vi "main OP500_V2.vi"() -> ()   [LabVIEW 2020]
uses:
  SubVI/OP500ZP_state.ctl
  <userlib>/Alex.vi/FGV.ctl
  <vilib>/QMT/GDataBase for MySQL(tm)/MySQL/public/controls/DateType.ctl
  VG/VG_progressBar.vi
  SubVI/CheminDeBase.vi
  <vilib>/Utility/error.llb/Error Cluster From Error Code.vi
  VG/PN.vi
  VG/PackType.vi
  VG/IS30%.vi
  VG/VG_branche.vi
  VG/Ubatt.vi
  VG/VG_BT3562.vi
  SubVI/OP500ZP_VGConf.vi
  <vilib>/QMT/GDataBase for MySQL(tm)/MySQL/MySQLConnector.lvclass
panel:
  in  "?":bool
  out "N° Révision":u32
  out "IS30% ?":bool
  out "BDD":T1
  out "VISA OUT":T2
  out "progression":u8(slide) scale=0.0..100.0
  out "PN":string
  out "errout 2":errorcluster={"status"=TRUE, "code"=0, "source"="PCAN_CHANNEL ILLEGAL"} caption="errout"
  out "errout":errorcluster caption="sortie d'erreur"
  out "STOP":bool
  out "TOP":string
  out "DRAW":picture
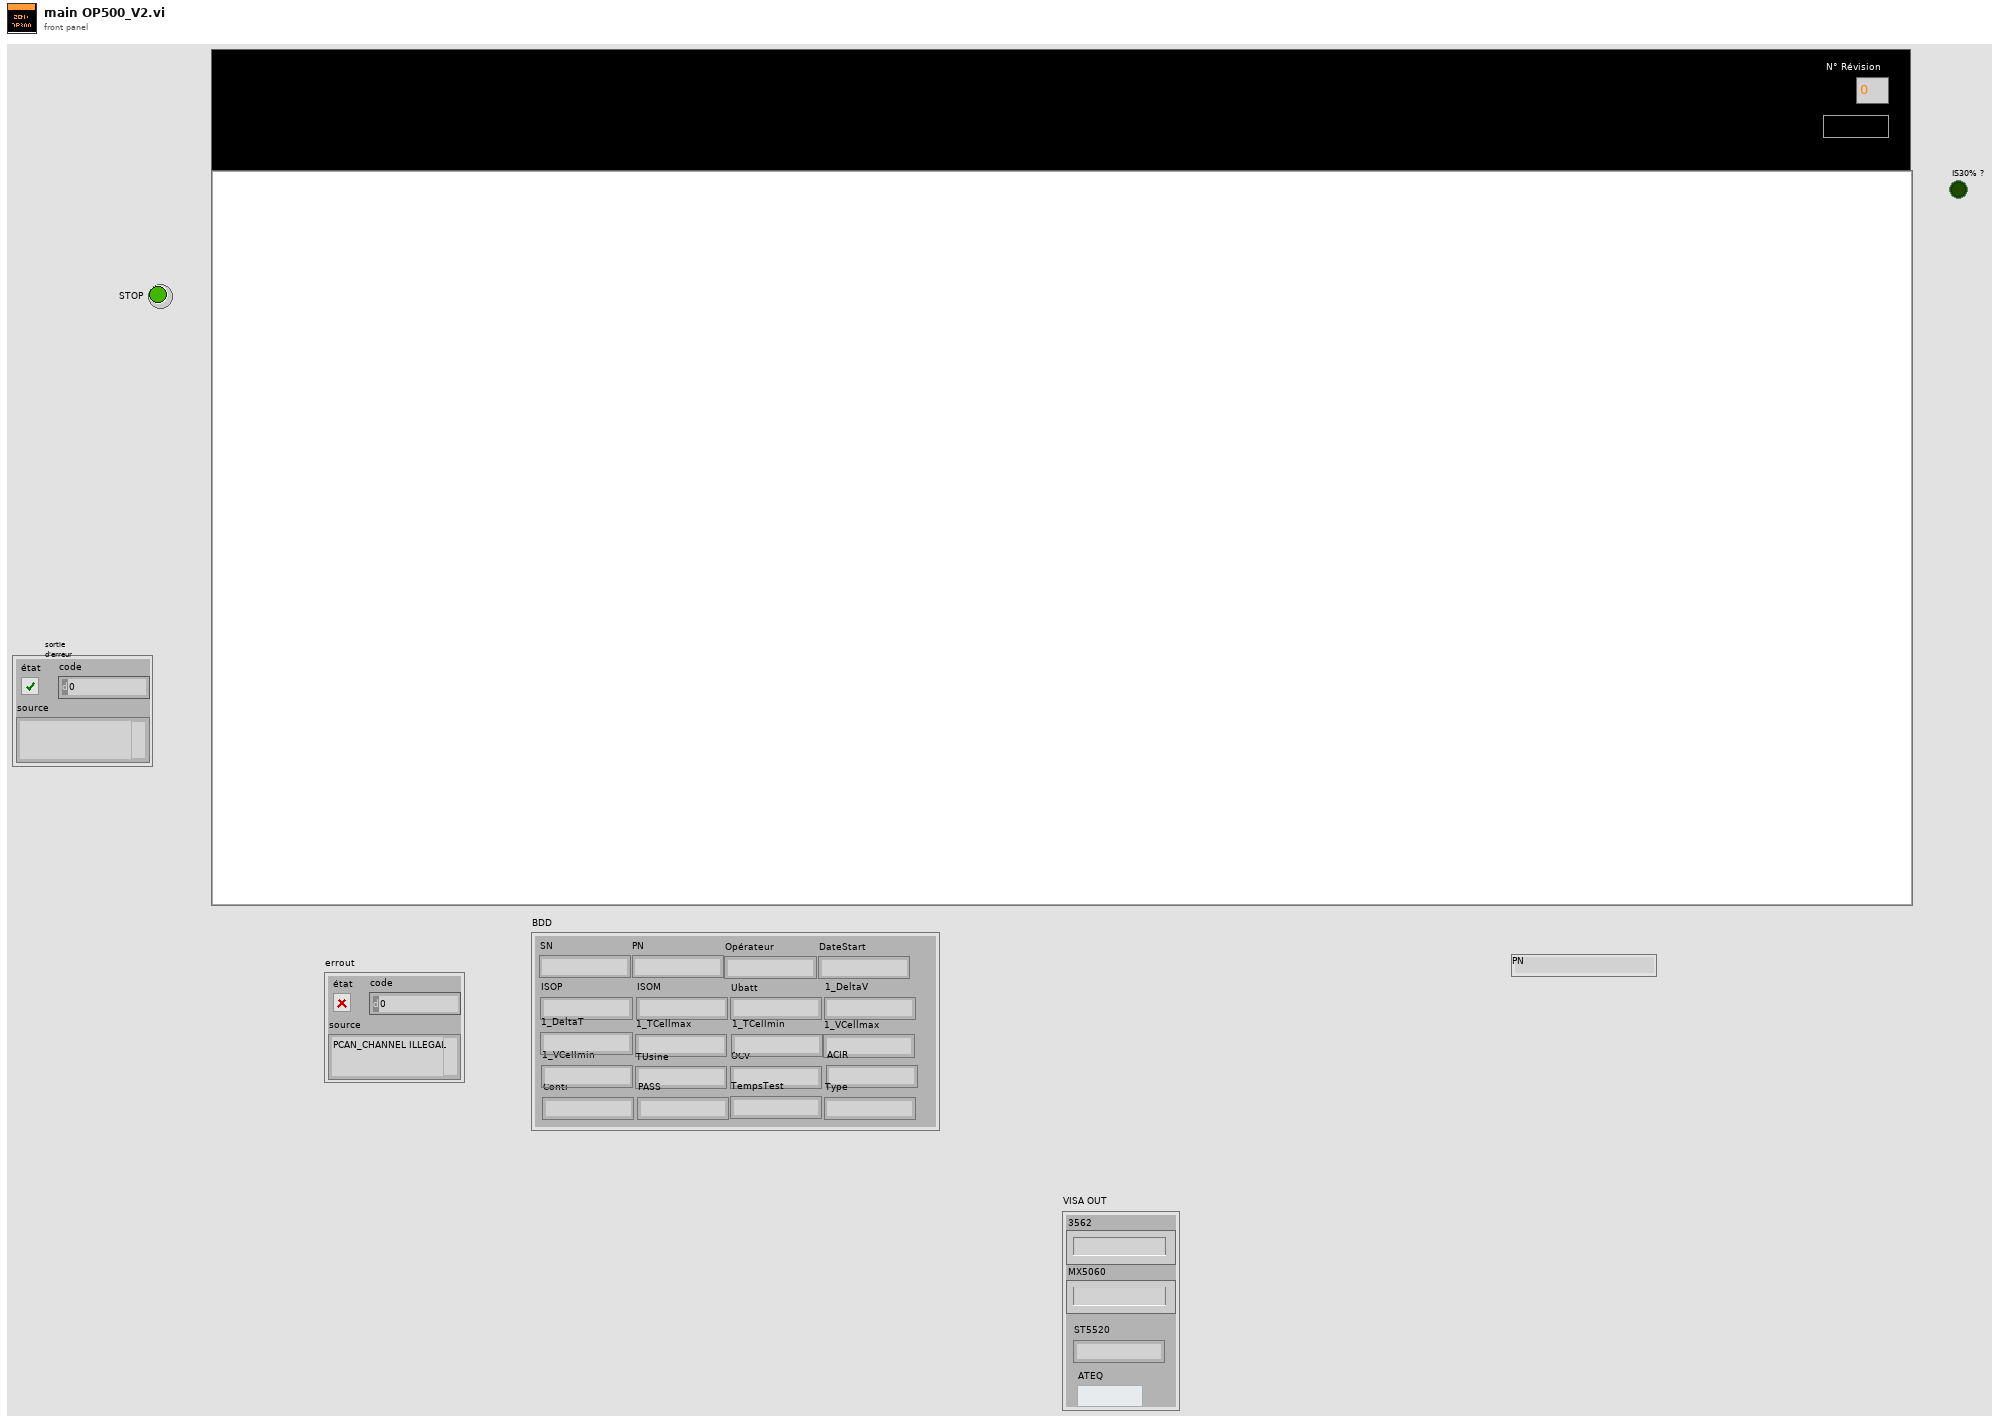
[diagram p1: front panel]
types:
  T1 = cluster{"SN":string, "PN":string, "Opérateur":string, "DateStart":string, "ISOP":string, "ISOM":string, "Ubatt":string, "1_DeltaV":string, "1_DeltaT":string, "1_TCellmax":string, "1_TCellmin":string, "1_VCellmax":string, "1_VCellmin":string, "TUsine":string, "OCV":string, "ACIR":string, "Conti":string, "PASS":string, "TempsTest":string, "Type":string}
  T2 = cluster{"3562":string, "MX5060":string, "ST5520":string, "ATEQ":string}
  T3 = cluster{"PN":string, "Sealing":string, "Opérateur":string, "Conti":string, "OCV":string, "ISOP":string, "ISOM":string, "1_TCellmin":string, "1_TCellmax":string, "1_VCellmin":string, "1_VCellmax":string, "1_Nbmodule":string, "2_TCellmin":string, "2_TCellmax":string, "2_VCellmin":string, "2_VCellmax":string, "2_Nbmodule":string, "Résultat final":string, "Résultat final 2":string, "Résultat final 3":string}
  T4 = cluster{"3562":string, "MX5060":string, "ST5520":string, string}
  T5 = typedef "OP500ZP_state.ctl" = enum16{"Null", "Demarrage", "Init", "Scan", "Iso", "Softs", "MCU", "OCVACIR", "Conti", "DTC", "DataDyn", "DataDyn2", "Crash", "Next", "Comext"}
  T6 = typedef "FGV.ctl" = enum16{"GET", "SET", "RAZ"}
  T7 = typedef "MySQLVIEW.lvlib/MySQLConnector.lvclass/DateType.ctl" = enum16{"DATETIME", "DATE", "TIMESTAMP", "TIME", "YEAR (2 digits)", "YEAR (4 digits)"}
  T8 = cluster{string, string, string, string, string, string, string, string}
  T9 = typedef "OP500ZP_state.ctl" = enum16{"Null", "Demarrage", "Init", "Scan", "Montage", "Conti", "OCV", "Iso", "Softs", "Vpack", "DataDyn", "Dessouter", "DataDyn2", "Demontage", "Crash", "Next", "Sealing", "Comext"}
  T10 = cluster{"Chaîne":string, "Chaîne":string, "Chaîne":string, "Chaîne":string, "Chaîne":string, "Chaîne":string, "Chaîne":string, "Chaîne 2":string}
  T11 = typedef "imagedata.ctl" = cluster{"image type":i32, "image depth":i32, "image":u8[], "mask":u8[], "colors":u32[], "Rectangle":cluster{"left":i16, "top":i16, "right":i16, "bottom":i16}}
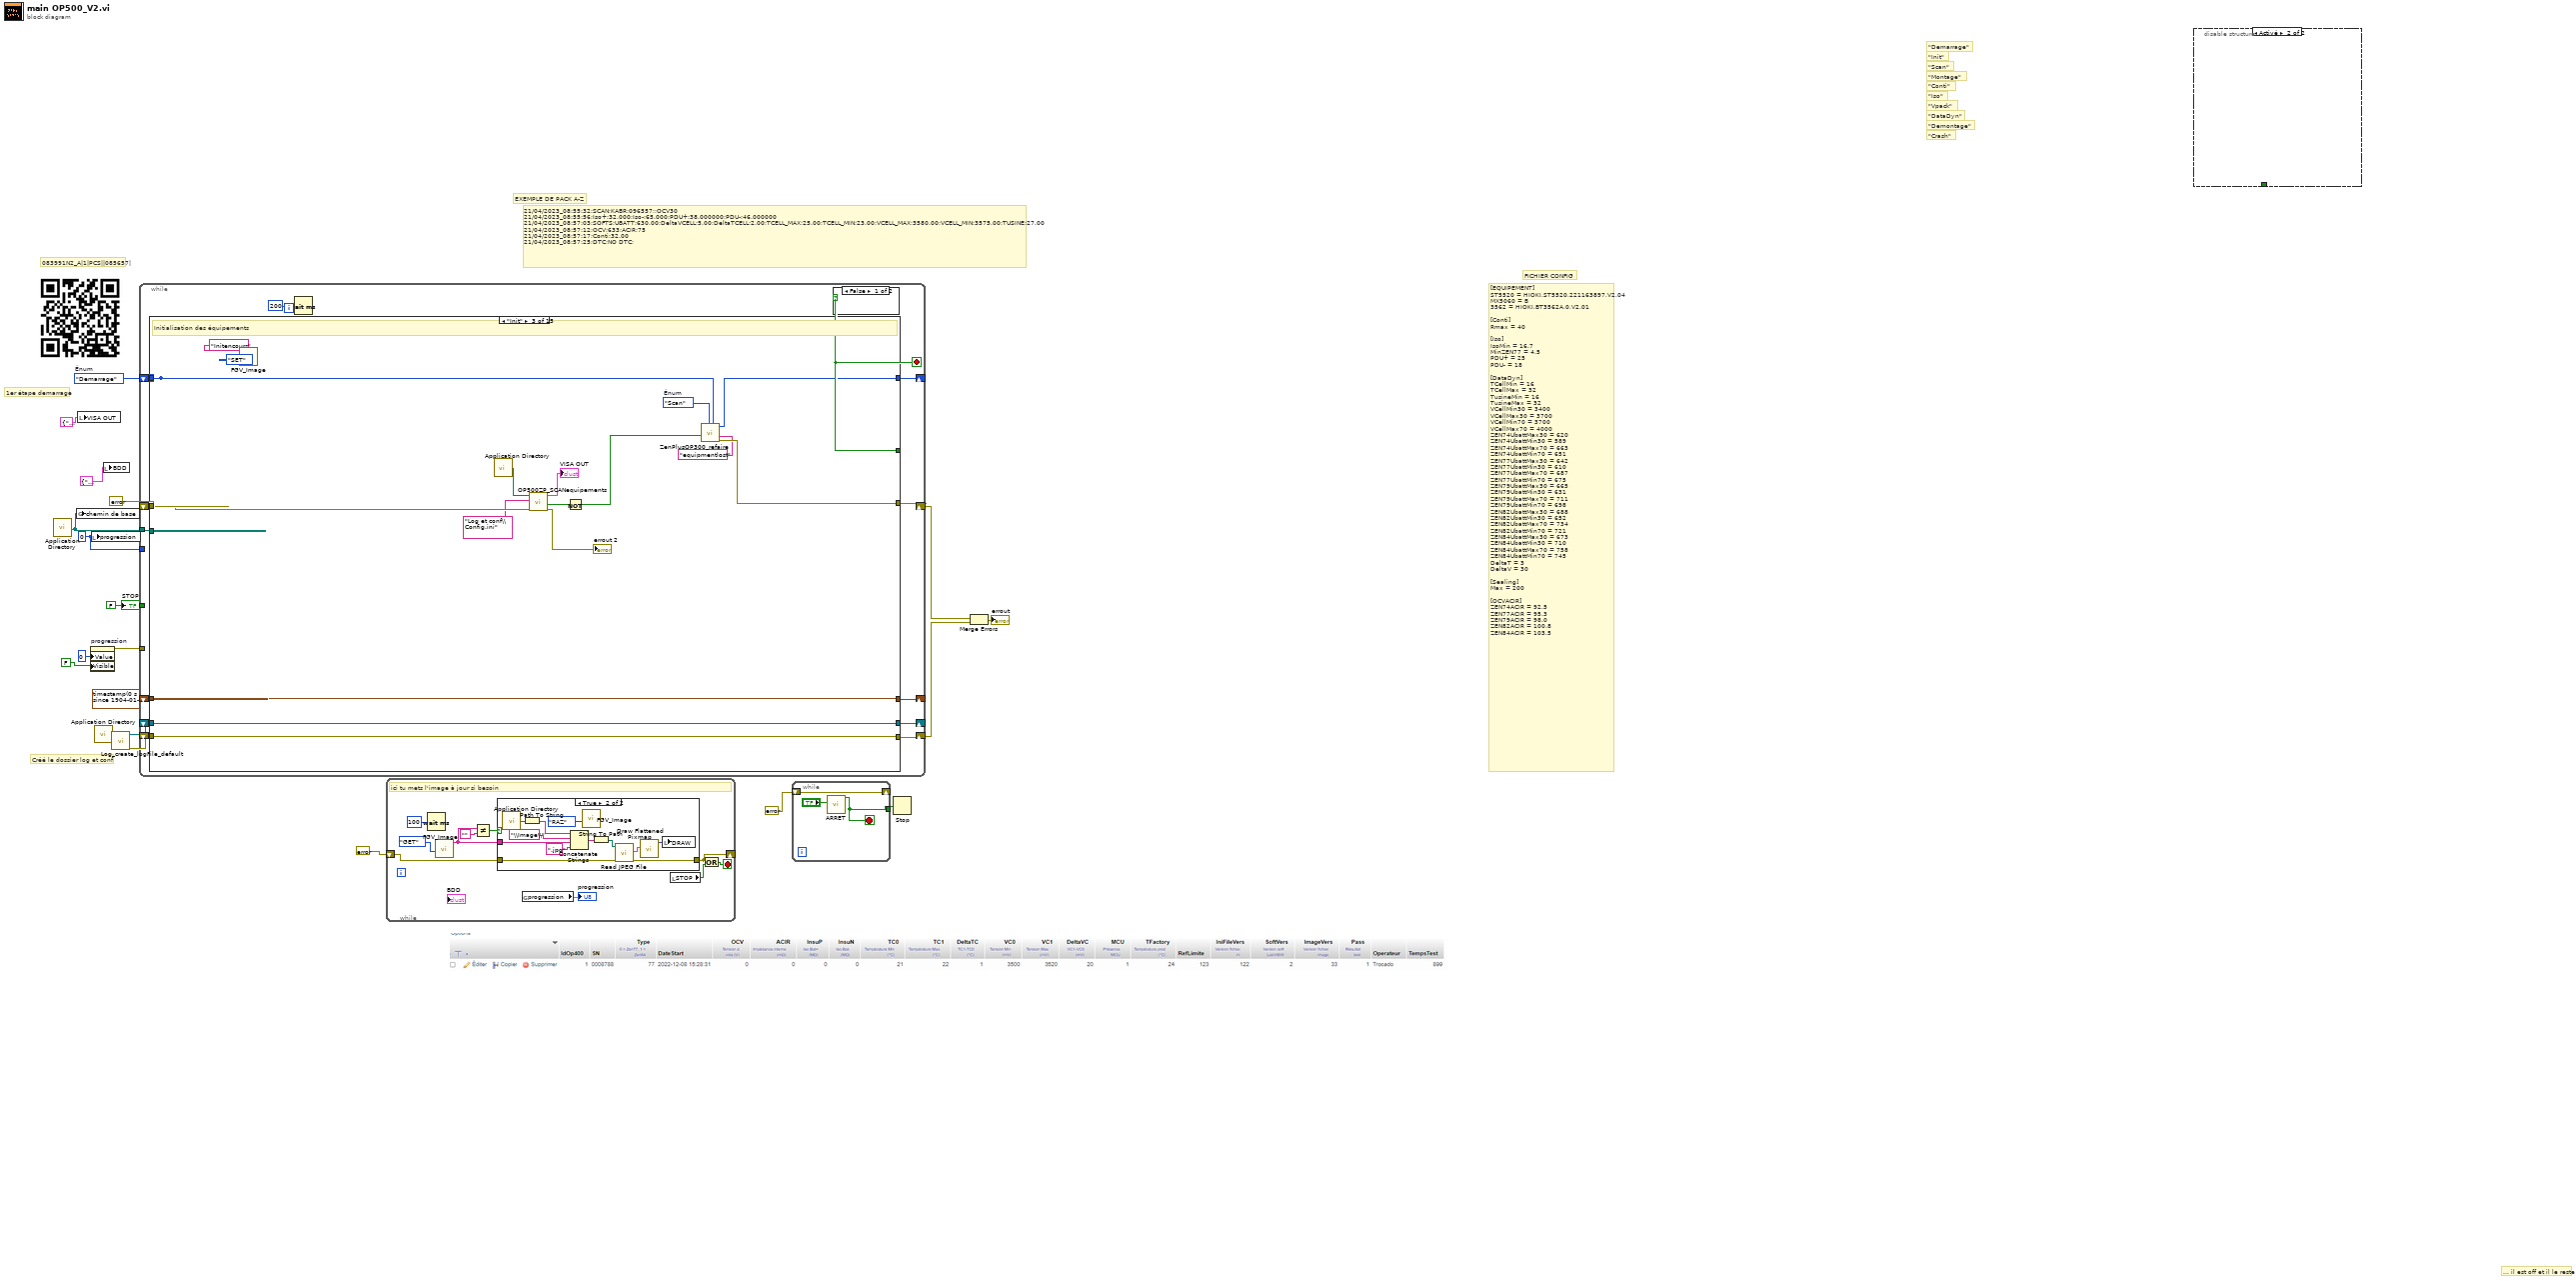
[diagram p0: block diagram]
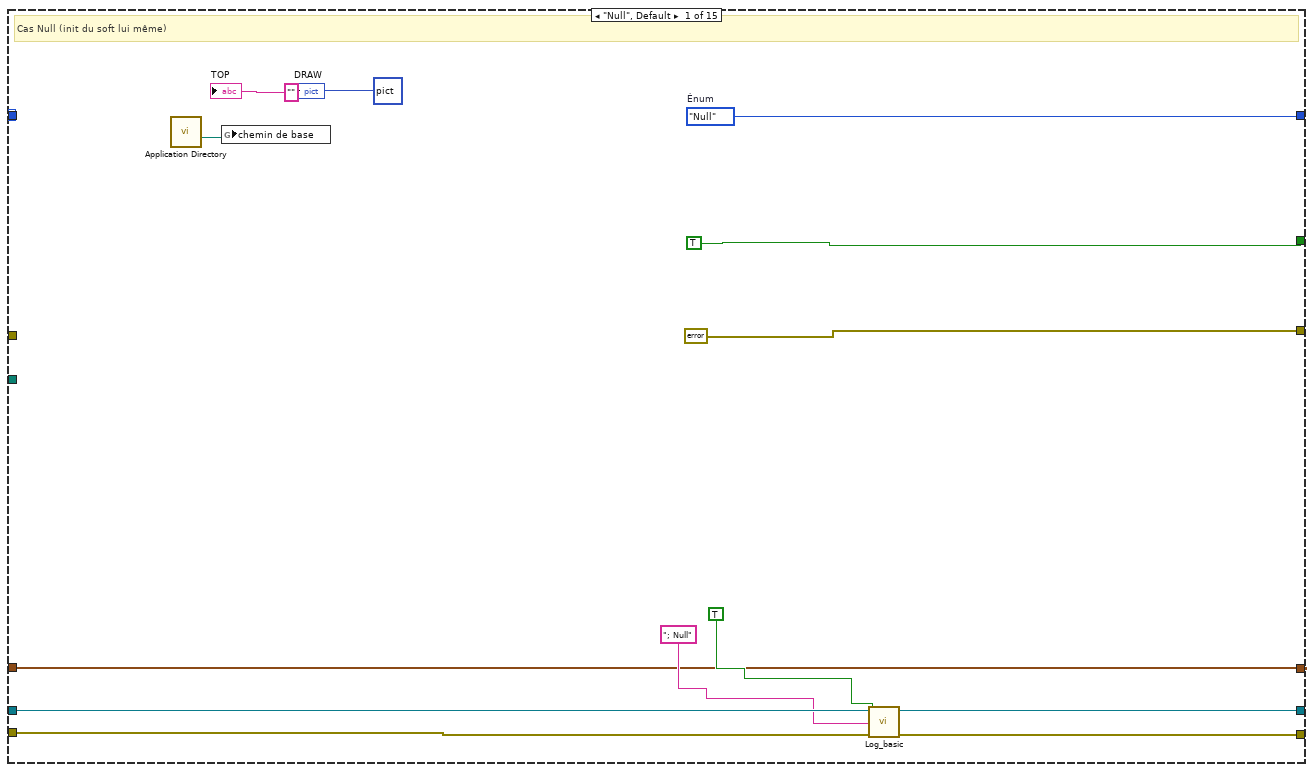
[diagram p2: hidden frame]
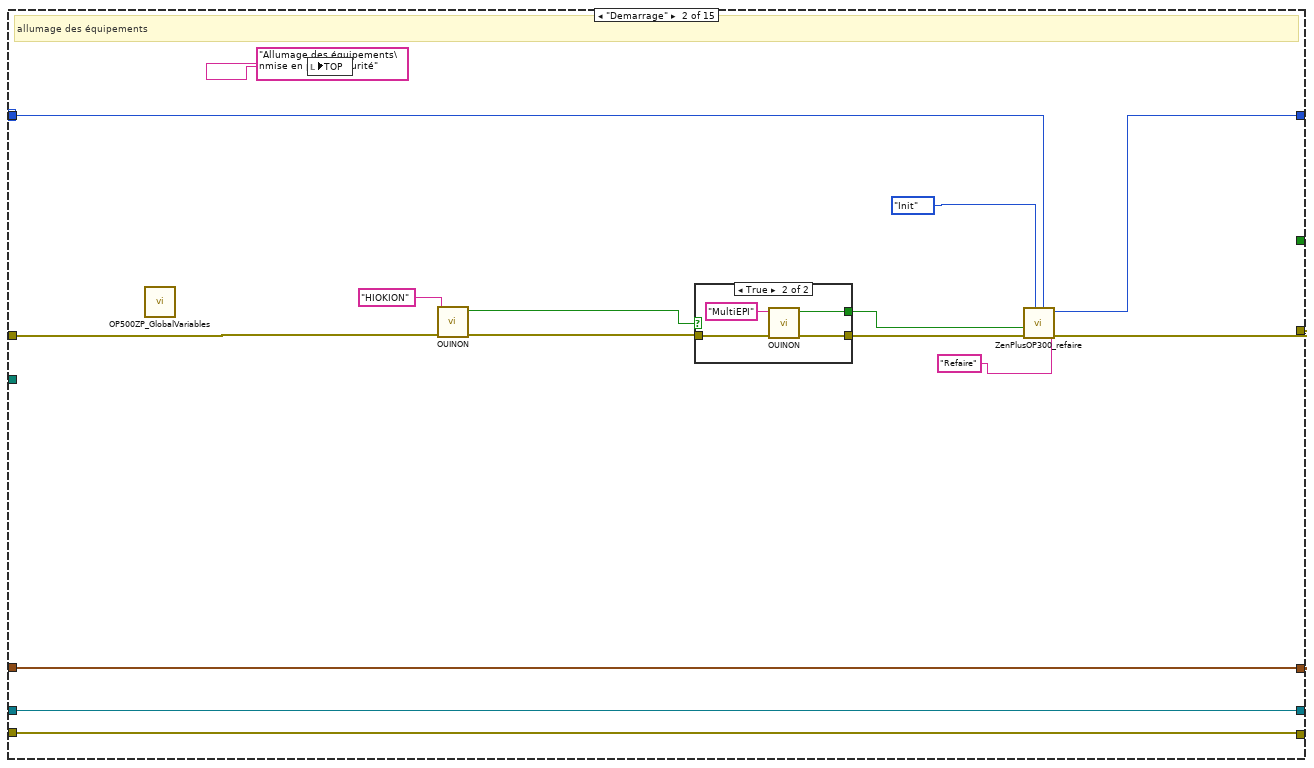
[diagram p3: hidden frame]
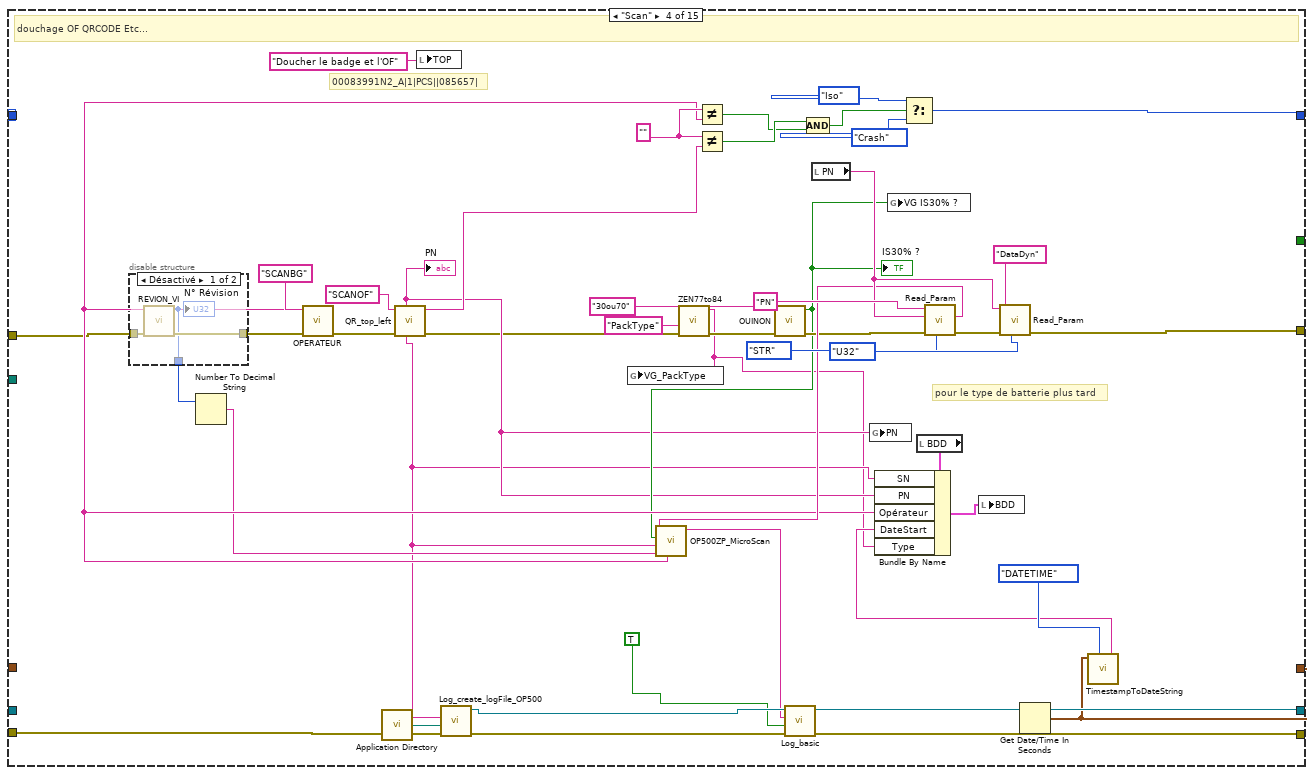
[diagram p5: hidden frame]
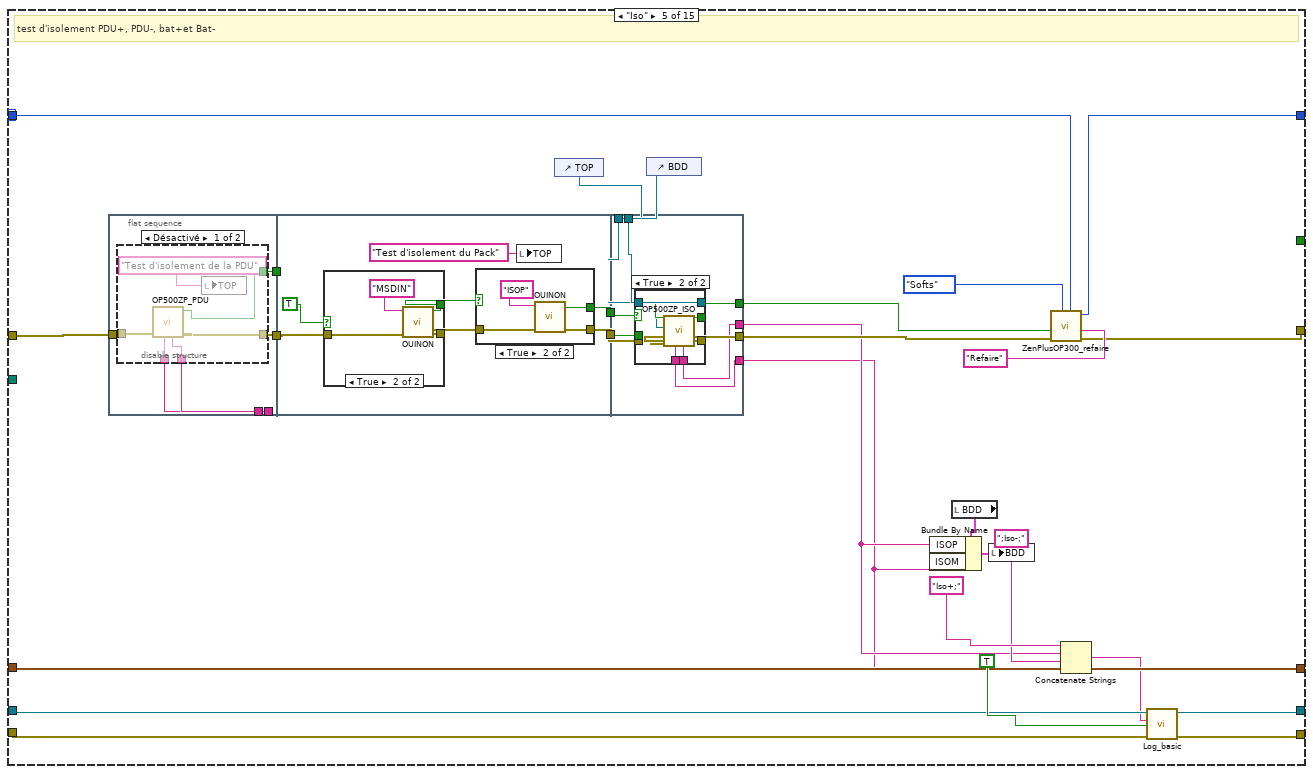
[diagram p7: hidden frame]
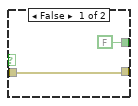
[diagram p9: hidden frame]
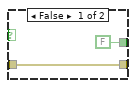
[diagram p10: hidden frame]
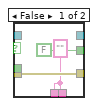
[diagram p11: hidden frame]
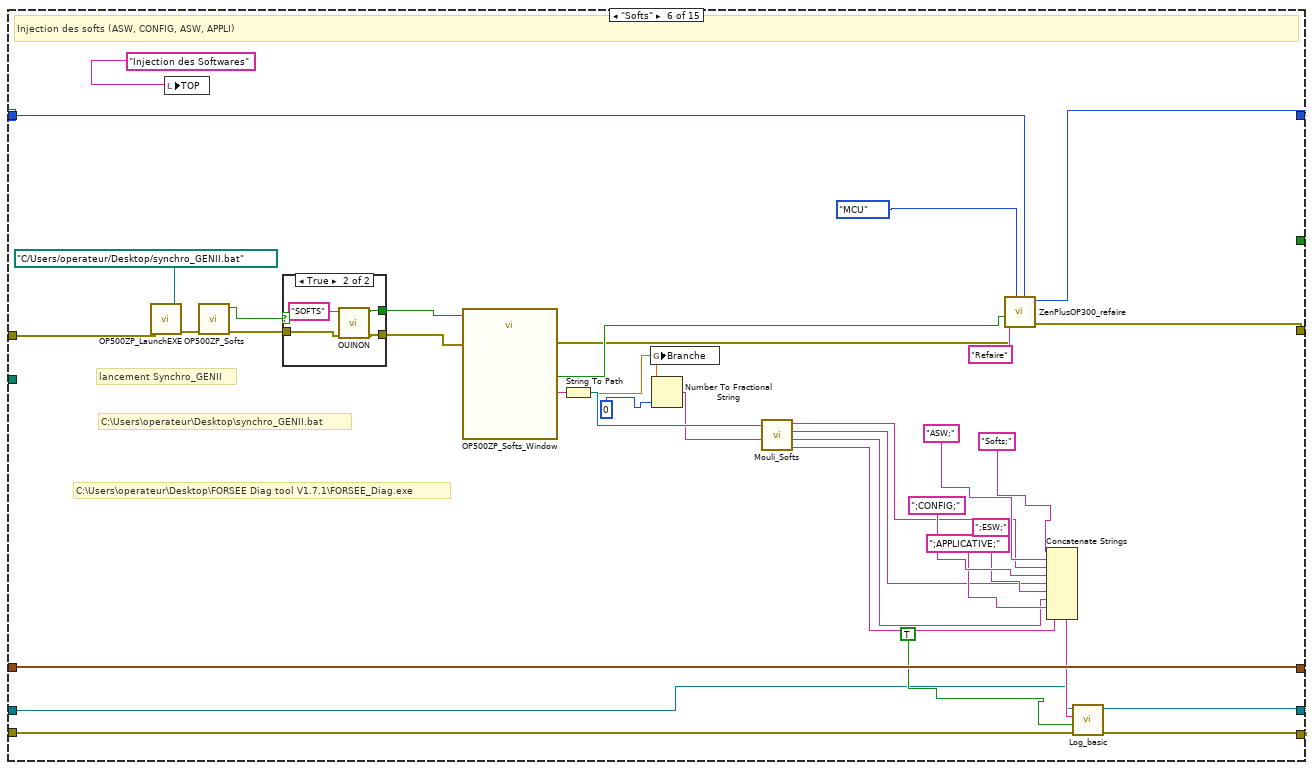
[diagram p12: hidden frame]
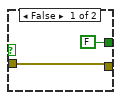
[diagram p13: hidden frame]
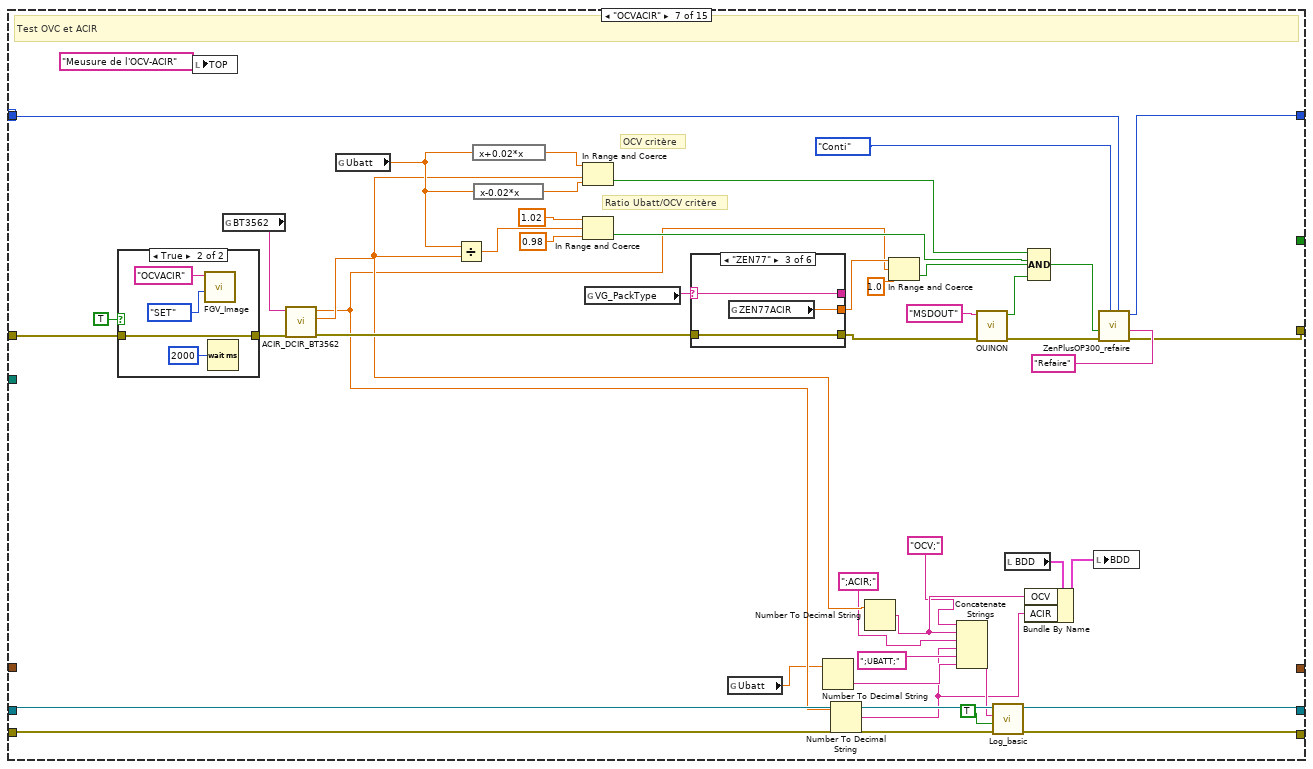
[diagram p14: hidden frame]
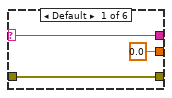
[diagram p16: hidden frame]
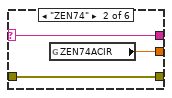
[diagram p17: hidden frame]
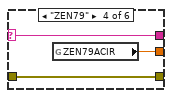
[diagram p18: hidden frame]
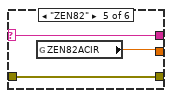
[diagram p19: hidden frame]
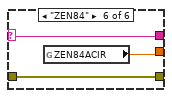
[diagram p20: hidden frame]
diagram:
  w10 = u8 0 ("progression")
  w5 = OP500ZP_state."Demarrage"  # Énum
  w16 = FALSE ("STOP")
  # "083991N2_A|1|PCS||085657|"
  # "EXEMPLE DE PACK A-Z"
  # "21/04/2023_08:55:32;SCAN;KABR;096557;;OCV30\n21/04/2023_08:55:56;Iso+;32.000;Iso-;65.000;PDU+;38.000000;PDU-;46.000000\n21/04/2023_08:57:03;SOFTS;UBATT;630.00;DeltaVCELL;5.00;DeltaTCELL;2.00;TCELL_MAX;25.00;TCELL_MIN;23.00;VCELL_MAX;3580.00;VCELL_MIN;3575.00;TUSINE;27.00\n21/04/2023_08:57:12;OCV;633;ACIR;75\n21/04/2023_08:57:17;Conti;32.00\n21/04/2023_08:57:25;DTC;NO DTC;"
  # "FICHIER CONFIG"
  # "[EQUIPEMENT]\nST5520 = HIOKI,ST5520,221163897,V2.04\t\nMX5060 = B\n3562 = HIOKI,BT3562A,0,V2.01\n\n[Conti]\nRmax = 40\n\n[Iso]\nIsoMin = 16.7\nMinZEN77 = 4.5\nPDU+ = 25\nPDU- = 18\n\n[DataDyn]\nTCellMin = 16\nTCellMax = 32\nTusineMin = 16\nTusineMax = 32\nVCellMin30 = 3400\nVCellMax30 = 3700\nVCellMin70 = 3700\nVCellMax70 = 4000\nZEN74UbattMax30 = 620\nZEN74UbattMin30 = 589\nZEN74UbattMax70 = 663\nZEN74UbattMin70 = 651\nZEN77UbattMax30 = 642\nZEN77UbattMin30 = 610\nZEN77UbattMax70 = 687\nZEN77UbattMin70 = 675\nZEN79UbattMax30 = 665\nZEN79UbattMin30 = 631\nZEN79UbattMax70 = 711\nZEN79UbattMin70 = 698\nZEN82UbattMax30 = 688\nZEN82UbattMin30 = 652\nZEN82UbattMax70 = 734\nZEN82UbattMin70 = 721\nZEN84UbattMax30 = 673\nZEN84UbattMin30 = 710\nZEN84UbattMax70 = 758\nZEN84UbattMin70 = 745\nDeltaT = 3\nDeltaV = 30\n\n[Sealing]\nMax = 200\n\n[OCVACIR]\nZEN74ACIR = 92.5\nZEN77ACIR = 95.3\nZEN79ACIR = 98.0\nZEN82ACIR = 100.8\nZEN84ACIR = 103.5"
  # "Créé le dossier log et conf"
  # "1er étape demarrage"
  # "\"Crash\""
  # "\"Demontage\""
  # "\"DataDyn\""
  # "\"Iso\""
  # "\"Montage\""
  # "\"Scan\""
  # "\"Init\""
  # "\"Demarrage\""
  # "\"Conti\""
  # "\"Vpack\""
  # "... il est off et il le reste"
  n1 = call <vilib>:"Application Directory.vi"() -> ("Application Directory"=w15:path)
  n2 = global write "CheminDeBase.vi" "chemin de base"(w15) -> ()
  n3 = local write "VISA OUT"(T4 {"3562"="", "MX5060"="", "ST5520"="", ""} ("VISA OUT")) -> ()
  n4 = property on="progression" class="Slide (strict)"("Value"=u8 0 ("progression"), "Visible"=FALSE) -> (error out=w8:errorcluster)  [unwired: 2 in, 1 out]
  n5 = local write "progression"(w10) -> ()
  n6 = call <vilib>:"Application Directory.vi"() -> ("Application Directory"=w13:path)
  n7 = local write "BDD"(T3 {"PN"="0", "Sealing"="0", "Opérateur"="0", "Conti"="0", "OCV"="0", "ISOP"="0", "ISOM"="0", "1_TCellmin"="0", "1_TCellmax"="0", "1_VCellmin"="0", "1_VCellmax"="0", "1_Nbmodule"="0", "2_TCellmin"="0", "2_TCellmax"="0", "2_VCellmin"="0", "2_VCellmax"="0", "2_Nbmodule"="0", "Résultat final"="0", "Résultat final 2"="0", "Résultat final 3"="0"} ("Cluster")) -> ()
  n8 = call <userlib>:"Log_create_logFile_default.vi"("appdir"=w13) -> ("errout"=w14:errorcluster, "Fichier à flux d'octets en sortie"=w17:refnum<file>)  [unwired: 9 in]
  n9 = while {
    shift-right: [w32] -> w19
    shift-left: errorcluster {"status"=FALSE, "code"=0, "source"=""} ("error out") -> [w24]
    shift-right: [w28] -> w18
    shift-left: w14 -> [w31]
    shift-right: [w29] -> _
    shift-left: w17 -> [w30]
    tunnel: w15 -> [w27]
    tunnel: w16 -> [_]
    shift-right: [w25] -> _
    shift-left: timestamp(0 s since 1904-01-01) ("seconds since 1Jan1904") -> [w26]
    tunnel: w10 -> [_]
    tunnel: w8 -> [_]
    shift-right: [w23] -> _
    shift-left: w5 -> [w22]
    stop <- w21 stop-if-true
    n10 = case shown="\"Init\"" w22 {
      selector: w22 -> [_ w50 w80 _ _ w239 w291 w342 w395 _ w469 _ _ w594 w694]
      tunnel: w24 -> [_ w60 w74 w93 w146 w237 w255 w323 w376 w439 w461 w523 w555 w591 w691]
      tunnel: [errorcluster {"status"=FALSE, "code"=0, "source"=""} ("errin") w51 w81 w115 w144 w241 w290 w343 w396 w443 w462 w522 w558 w593 w696] -> w32
      tunnel: w31 -> [w42 w54 w84 w128 w159 w230 w287 w349 w389 w448 w465 w545 w578 w597 w703]
      tunnel: w30 -> [w43 w61 w83 _ w158 w228 w289 w348 w387 w447 w467 w546 w579 w596 w702]
      tunnel: [w40 w61 w83 w130 w157 w227 w288 w347 w386 w446 w463 _ _ w588 w700] -> w29
      tunnel: [w41 w54 w84 w131 w160 w229 w286 w346 w388 w445 w464 w524 w556 w595 w701] -> w28
      tunnel: [TRUE _ _ _ _ _ _ _ _ _ _ w547 _ _ _] -> w21
      tunnel: w27 -> [_ _ _ _ _ _ _ _ _ _ w468 _ _ w592 _]
      tunnel: w26 -> [w37 w59 w82 _ w156 w245 _ w345 w384 w427 w466 _ _ w589 w699]
      tunnel: [w37 w59 w82 w88 w156 w245 _ w345 w384 w427 w466 _ _ w590 w699] -> w25
      tunnel: [w34 w48 w78 w94 w141 w240 w275 w336 w393 w425 w460 OP500ZP_state."Crash" w557 w587 w693] -> w23
      tunnel: w22 -> [_ _ _ _ w142 _ _ _ _ _ _ _ _ _ _]
      frame "Null", Default {
        w34 = OP500ZP_state."Null"  # Énum
        # "Cas Null (init du soft lui même)"
        n11 = call <vilib>:"Application Directory.vi"() -> ("Application Directory"=w46:path)
        n12 = global write "CheminDeBase.vi" "chemin de base"(w46) -> ()
        n13 = call <userlib>:"Log_basic.vi"("errin"=w42, "date?"=TRUE, "chaîne"="; Null", "in"=w43) -> ("sortie d'erreur"=w41:errorcluster, "refnum en sortie"=w40:refnum<file>)  [unwired: 6 in]
        "DRAW" <- picture data[5B] ("DRAW")
        "TOP" <- "" ("TOP")
      }
      frame "Demarrage" {
        # "allumage des équipements"
        n14 = call "OP500ZP_GlobalVariables.vi"() -> ()  [unwired: 12 in]
        n15 = local write "TOP"("Allumage des équipements\nmise en place sécurité" ("TOP")) -> ()
        n16 = call "OUINON.vi"("errin"=w60, "image"="HIOKION") -> ("error out"=w55:errorcluster, "OUI/NON"=w56:bool)  [unwired: 8 in]
        n17 = case shown="True" w56 {
          selector: w56 -> [w63 _]
          tunnel: [w63 w67] -> w47
          tunnel: [w62 w66] -> w52
          tunnel: w55 -> [w62 w64]
          frame False {
          }
          frame True {
            n18 = call "OUINON.vi"("errin"=w64, "image"="MultiEPI" ("IN")) -> ("error out"=w66:errorcluster, "OUI/NON"=w67:bool)  [unwired: 8 in]
          }
        }
        n19 = call "ZenPlusOP300_refaire.vi"("image"="Refaire", "refaire"=w50, "casOK"=OP500ZP_state."Init", "errin"=w52, "test ok ?"=w47) -> ("errout"=w51:errorcluster, "Next"=w48:T5)  [unwired: 5 in]
      }
      frame "Init" {
        w77 = OP500ZP_state."Scan"  # Énum
        # "Initialisation des équipements"
        n20 = call <userlib>:"FGV_Image.vi"("Énum"=FGV."SET", "IN"="Initencours") -> ()  [unwired: 9 in, 1 out]
        n21 = call <vilib>:"Application Directory.vi"() -> ("Application Directory"=w72:path)
        n22 = call "OP500ZP_SCANequipements.vi"("Errin"=w74, "Chaîne"="Log et conf\\Config.ini", "pathin"=w72) -> ("ERROUT"=→"errout 2":errorcluster, "KO?"=w69:bool, "VISA OUT"=→"VISA OUT":T2)  [unwired: 6 in]
        n23 = Not(x=w69) -> (.not. x?=w68:bool)
        n24 = call "ZenPlusOP300_refaire.vi"("image"="equipmentlost", "refaire"=w80, "casOK"=w77, "test ok ?"=w68) -> ("errout"=w81:errorcluster, "Next"=w78:T5)  [unwired: 6 in]
      }
      frame "Scan" {
        w123 = "" ("x")
        # "pour le type de batterie plus tard"
        # "00083991N2_A|1|PCS||085657|"
        # "douchage OF QRCODE Etc..."
        n25 = disable-structure shown="Désactivé" {
          disable-tunnel: w93 -> [w134 _]
          disable-tunnel: [w133 _] -> w92
          disable-tunnel: [w132 _] -> w91
          frame Disabled {
            n26 = call "REVION_VI.vi"("ERRIN"=w134) -> ("ERROUT"=w133:errorcluster, "N° Révision"=w132:u32)  [unwired: 9 in]
            "N° Révision" <- w132
          }
          frame Enabled {
          }
        }
        n27 = Number To Decimal String(number=w91) -> (decimal integer string=w90:string)  [unwired: 1 in]
        n28 = call <userlib>:"OPERATEUR.vi"("errin"=w92, "IN"="SCANBG") -> ("error out"=w120:errorcluster, "Dataout"=w102:string)  [unwired: 8 in]
        n29 = call <vilib>:"Application Directory.vi"() -> ("Application Directory"=w129:path)
        n30 = call "QR_top_left.vi"("errin"=w120, "image"="SCANOF") -> ("error out"=w97:errorcluster, "Réponse"=w118:string, "SN"=w89:string, "PN"=w98:string)  [unwired: 5 in, 1 out]
        "PN" <- w98
        n31 = local write "TOP"("Doucher le badge et l'OF" ("TOP")) -> ()
        n32 = call "Log_create_logFile_OP500.vi"("errin"=w128, "toute l'expression"=w89, "Application Directory"=w129) -> ("sortie d'erreur"=w126:errorcluster, "Fichier à flux d'octets en sortie"=w127:refnum<file>)  [unwired: 7 in]
        n33 = call <userlib>:"ZEN77to84.vi"("errin"=w97, "image"="PackType") -> ("error out"=w96:errorcluster, "Réponse"=w85:string)  [unwired: 8 in]
        n34 = global write "PackType.vi" "VG_PackType"(w85) -> ()
        n35 = Not Equal?(x=w123, y=w102) -> (x != y?=w121:bool)
        n36 = Not Equal?(x=w123, y=w118) -> (x != y?=w122:bool)
        n37 = call "OUINON.vi"("errin"=w96, "image"="30ou70") -> ("error out"=w100:errorcluster, "OUI/NON"=w99:bool)  [unwired: 8 in]
        "IS30% ?" <- w99
        n38 = Compound Arithmetic op=AND ("Opérateur arithmétique")(w122, w121) -> (w108:bool)
        n39 = local read "PN"() -> (w111:string)
        n40 = global write "PN.vi" "PN"(w98) -> ()
        n41 = global write "IS30%.vi" "VG IS30% ?"(w99) -> ()
        n42 = Select ("Sélectionner")(t=OP500ZP_state."Iso" ("Énum"), s=w108, f=OP500ZP_state."Crash" ("cas faux")) -> (s? t:f=w94:T5)
        n43 = local read "BDD"() -> (w104:T1)
        n44 = call <userlib>:"Read_Param.vi"("Énum"=enum16{"STR", "DBL", "U32"}."STR", "errin"=w100, "section"=w111, "key"="PN") -> ("error out"=w114:errorcluster, "str"=w110:string)  [unwired: 3 in, 3 out]
        n45 = call "OP500ZP_MicroScan.vi"("Dataout"=w102, "Rev"=w90, "SN"=w89, "Oui"=w99, "str"=w110) -> ("Chaîne"=w125:string)  [unwired: 6 in]
        n46 = call <userlib>:"Log_basic.vi"("errin"=w126, "date?"=TRUE, "chaîne"=w125, "in"=w127) -> ("sortie d'erreur"=w131:errorcluster, "refnum en sortie"=w130:refnum<file>)  [unwired: 6 in]
        n47 = call <userlib>:"Read_Param.vi"("Énum"=enum16{"STR", "DBL", "U32"}."U32", "errin"=w114, "section"="DataDyn", "key"=w111) -> ("error out"=w115:errorcluster)  [unwired: 3 in, 4 out]
        n48 = Get Date/Time In Seconds() -> (seconds since 1Jan1904=w88:timestamp)
        n49 = call <vilib>:"TimestampToDateString.vi"("dateType"=DateType."DATETIME", "timestamp in"=w88) -> ("dateString"=w86:string)  [unwired: 8 in, 1 out]
        n50 = Bundle By Name(cluster=w104, "SN"=w89, "PN"=w98, "Opérateur"=w102, "DateStart"=w86, "Type"=w85) -> (w103:T1)
        n51 = local write "BDD"(w103) -> ()
      }
      frame "Iso" {
        # "test d'isolement PDU+, PDU-, bat+et Bat-"
        n52 = flat-sequence {
          tunnel: [w164] -> w148
          tunnel: [w165] -> w147
          tunnel: w146 -> [w166]
          tunnel: [w163] -> _
          tunnel: [w162] -> _
          tunnel: [w179] -> w150
          tunnel: [w178] -> w149
          tunnel: w148 -> [_]
          tunnel: w147 -> [w173]
          tunnel: [w199] -> w140
          tunnel: [w192] -> w135
          tunnel: [w193] -> w136
          tunnel: w152 -> [w197]
          tunnel: w151 -> [w196]
          tunnel: w150 -> [w198]
          tunnel: w149 -> [w195]
          tunnel: [w194] -> w139
          frame #0 {
            n53 = disable-structure shown="Désactivé" {
              disable-tunnel: w166 -> [w172 _]
              disable-tunnel: [w171 _] -> w165
              disable-tunnel: [w170 _] -> w164
              disable-tunnel: [w169 _] -> w163
              disable-tunnel: [w168 _] -> w162
              frame Disabled {
                n54 = call "OP500ZP_PDU.vi"("errin"=w172) -> ("errout"=w171:errorcluster, "PASS?"=w170:bool, "ISO_PDU-"=w169:string, "ISO_PDU+"=w168:string)  [unwired: 7 in]
                n55 = local write "TOP"("Test d'isolement de la PDU" ("TOP")) -> ()
              }
              frame Enabled {
              }
            }
          }
          frame #1 {
            n56 = case shown="True" TRUE {
              tunnel: w173 -> [w181 w185]
              tunnel: [w181 w184] -> w177
              tunnel: [FALSE ("OUI/NON") w182] -> w175
              frame False {
              }
              frame True {
                n57 = call "OUINON.vi"("errin"=w185, "image"="MSDIN") -> ("error out"=w184:errorcluster, "OUI/NON"=w182:bool)  [unwired: 8 in]
              }
            }
            n58 = case shown="True" w175 {
              tunnel: [w186 w191] -> w179
              tunnel: [FALSE ("OUI/NON") w190] -> w178
              tunnel: w177 -> [w186 w188]
              frame False {
              }
              frame True {
                n59 = call "OUINON.vi"("errin"=w188, "image"="ISOP" ("IN")) -> ("error out"=w191:errorcluster, "OUI/NON"=w190:bool)  [unwired: 8 in]
              }
            }
            n60 = local write "TOP"("Test d'isolement du Pack" ("TOP")) -> ()
          }
          frame #2 {
            n61 = case shown="True" w195 {
              tunnel: [w202 w209] -> w199
              tunnel: w198 -> [w202 w208]
              tunnel: w195 -> [_ w207]
              tunnel: w197 -> [_ _]
              tunnel: w196 -> [_ w206]
              tunnel: [FALSE ("Booléen") w205] -> w194
              tunnel: [w200 w204] -> w193
              tunnel: [w200 w203] -> w192
              frame False {
                w200 = "" ("Chaîne")
              }
              frame True {
                n62 = call "OP500ZP_ISO.vi"("entrée d'erreur (pas d'erreur)"=w208, "Oui"=w207, "reference en entrée"=w206) -> ("sortie d'erreur"=w209:errorcluster, "Booléen"=w205:bool, "ISOP"=w204:string, "ISOM"=w203:string)  [unwired: 5 in]
              }
            }
          }
        }
        n63 = control-ref of="TOP"() -> (w151:refnum<vi>)
        n64 = control-ref of="BDD"() -> (w152:refnum<vi>)
        n65 = local read "BDD"() -> (w138:T1)
        n66 = Bundle By Name(cluster=w138, "ISOP"=w136, "ISOM"=w135) -> (w137:T1)
        n67 = local write "BDD"(w137) -> ()
        n68 = call "ZenPlusOP300_refaire.vi"("image"="Refaire", "refaire"=w142, "casOK"=OP500ZP_state."Softs", "errin"=w140, "test ok ?"=w139) -> ("errout"=w144:errorcluster, "Next"=w141:T5)  [unwired: 5 in]
        n69 = Concatenate Strings("Iso+;" ("chaîne"), w136, ";Iso-;" ("chaîne"), w135) -> (w153:string)
        n70 = call <userlib>:"Log_basic.vi"("errin"=w159, "date?"=TRUE, "chaîne"=w153, "in"=w158) -> ("sortie d'erreur"=w160:errorcluster, "refnum en sortie"=w157:refnum<file>)  [unwired: 6 in]
      }
      frame "Softs" {
        # "C:\\Users\\operateur\\Desktop\\FORSEE Diag tool V1.7.1\\FORSEE_Diag.exe"
        # "C:\\Users\\operateur\\Desktop\\synchro_GENII.bat"
        # "lancement Synchro_GENII"
        # "Injection des softs (ASW, CONFIG, ASW, APPLI)"
        n71 = call "OP500ZP_LaunchEXE.vi"("errin"=w237, "Application à lancer"=path "C:/Users/operateur/Desktop/synchro_GENII.bat") -> ("error out"=w244:errorcluster)  [unwired: 7 in]
        n72 = local write "TOP"("Injection des Softwares" ("TOP")) -> ()
        n73 = call "OP500ZP_Softs.vi"("errin"=w244) -> ("errout"=w217:errorcluster, "OUI/NON"=w214:bool)  [unwired: 9 in]
        n74 = case shown="True" w214 {
          tunnel: w217 -> [w246 w251]
          tunnel: [w246 w250] -> w216
          tunnel: [FALSE ("OUI/NON") w249] -> w215
          frame False {
          }
          frame True {
            n75 = call "OUINON.vi"("errin"=w251, "image"="SOFTS") -> ("error out"=w250:errorcluster, "OUI/NON"=w249:bool)  [unwired: 8 in]
          }
        }
        n76 = call "OP500ZP_Softs_Window.vi"("Enable"=w215, "error in (no error)"=w216) -> ("Répertoire softs :"=w236:string, "n° Branche"=w212:dbl, "OK"=w213:bool, "error out"=w211:errorcluster)  [unwired: 14 in]
        n77 = String To Path(string=w236) -> (path=w235:path)
        n78 = global write "VG_branche.vi" "Branche"(w212) -> ()
        n79 = Number To Fractional String(number=w212, precision (6)=i16 0 ("précision (6)")) -> (F-format string=w234:string)  [unwired: 2 in]
        n80 = call "Mouli_Softs.vi"("Branche"=w234, "chemin"=w235) -> ("APPL"=w219:string, "ESW"=w220:string, "CONFIG"=w221:string, "ASW"=w222:string)  [unwired: 6 in]
        n81 = call "ZenPlusOP300_refaire.vi"("image"="Refaire", "refaire"=w239, "casOK"=OP500ZP_state."MCU", "errin"=w211, "test ok ?"=w213) -> ("errout"=w241:errorcluster, "Next"=w240:T5)  [unwired: 5 in]
        n82 = Concatenate Strings("Softs;" ("chaîne"), "ASW;" ("chaîne"), w222, ";CONFIG;" ("chaîne"), w221, ";ESW;" ("chaîne"), w220, ";APPLICATIVE;" ("chaîne"), w219) -> (w233:string)
        n83 = call <userlib>:"Log_basic.vi"("errin"=w230, "date?"=TRUE, "chaîne"=w233, "in"=w228) -> ("sortie d'erreur"=w229:errorcluster, "refnum en sortie"=w227:refnum<file>)  [unwired: 6 in]
      }
      frame "OCVACIR" {
        # "Ratio Ubatt/OCV critère"
        # "OCV critère"
        # "Test OVC et ACIR"
        n84 = case shown="True" TRUE {
          tunnel: [w297 w299] -> w259
          tunnel: w255 -> [w297 w299]
          frame False {
          }
          frame True {
            n85 = call <userlib>:"FGV_Image.vi"("Énum"=FGV."SET", "IN"="OCVACIR") -> ()  [unwired: 9 in, 1 out]
            n86 = Wait (ms)(milliseconds to wait=u32 2000 ("attente (ms)")) -> ()  [unwired: 1 out]
          }
        }
        n87 = local write "TOP"("Meusure de l'OCV-ACIR" ("TOP")) -> ()
        n88 = global read "VG_BT3562.vi" "BT3562"() -> (w258:string)
        n89 = call <instrlib>:"ACIR_DCIR_BT3562.vi"("errin"=w259, "VISA"=w258) -> ("sortie d'erreur"=w267:errorcluster, "V"=w266:dbl, "R"=w265:dbl)  [unwired: 4 in, 2 out]
        n90 = global read "Ubatt.vi" "Ubatt"() -> (w282:dbl)
        n91 = Divide(x=w282, y=w266) -> (x/y=w281:dbl)
        n92 = expression code="x+0.02*x"(w282) -> (w283:dbl)
        n93 = expression code="x-0.02*x"(w282) -> (w284:dbl)
        n94 = In Range and Coerce(upper limit=w283, x=w266, lower limit=w284) -> (In Range?=w278:bool)  [unwired: 1 out]
        n95 = In Range and Coerce(upper limit=1.02 ("limite supérieure"), x=w281, lower limit=0.98 ("limite inférieure")) -> (In Range?=w277:bool)  [unwired: 1 out]
        n96 = global read "PackType.vi" "VG_PackType"() -> (w285:string)
        n97 = case shown="\"ZEN77\"" w285 {
          selector: w285 -> [w304 w307 w310 w313 w316 w319]
          tunnel: [w304 w307 w310 w313 w316 w319] -> _
          tunnel: [0.0 ("ZEN84ACIR") w306 w309 w312 w315 w318] -> w274
          tunnel: [w302 w305 w308 w311 w314 w317] -> w270
          tunnel: w267 -> [w302 w305 w308 w311 w314 w317]
          frame Default {
          }
          frame "ZEN74" {
            n98 = global read "OP500ZP_VGConf.vi" "ZEN74ACIR"() -> (w306:dbl)
          }
          frame "ZEN77" {
            n99 = global read "OP500ZP_VGConf.vi" "ZEN77ACIR"() -> (w309:dbl)
          }
          frame "ZEN79" {
            n100 = global read "OP500ZP_VGConf.vi" "ZEN79ACIR"() -> (w312:dbl)
          }
          frame "ZEN82" {
            n101 = global read "OP500ZP_VGConf.vi" "ZEN82ACIR"() -> (w315:dbl)
          }
          frame "ZEN84" {
            n102 = global read "OP500ZP_VGConf.vi" "ZEN84ACIR"() -> (w318:dbl)
          }
        }
        n103 = global read "Ubatt.vi" "Ubatt"() -> (w257:dbl)
        n104 = Number To Decimal String(number=w257) -> (decimal integer string=w253:string)  [unwired: 1 in]
        n105 = Number To Decimal String(number=w265) -> (decimal integer string=w252:string)  [unwired: 1 in]
        n106 = Number To Decimal String(number=w266) -> (decimal integer string=w292:string)  [unwired: 1 in]
        n107 = In Range and Coerce(upper limit=w274, x=w265, lower limit=1.0 ("limite inférieure")) -> (In Range?=w272:bool)  [unwired: 1 out]
        n108 = Concatenate Strings("OCV;" ("chaîne"), w292, ";ACIR;" ("chaîne"), w252, ";UBATT;" ("chaîne"), w253) -> (w263:string)
        n109 = call "OUINON.vi"("errin"=w270, "image"="MSDOUT" ("IN")) -> ("error out"=w269:errorcluster, "OUI/NON"=w260:bool)  [unwired: 8 in]
        n110 = call <userlib>:"Log_basic.vi"("errin"=w287, "date?"=TRUE, "chaîne"=w263, "in"=w289) -> ("sortie d'erreur"=w286:errorcluster, "refnum en sortie"=w288:refnum<file>)  [unwired: 6 in]
        n111 = local read "BDD"() -> (w294:T1)
        n112 = Bundle By Name(cluster=w294, "OCV"=w292, "ACIR"=w252) -> (w293:T1)
        n113 = Compound Arithmetic op=AND ("Opérateur arithmétique")(w278, w277, w272, w260) -> (w271:bool)
        n114 = local write "BDD"(w293) -> ()
        n115 = call "ZenPlusOP300_refaire.vi"("image"="Refaire", "refaire"=w291, "casOK"=OP500ZP_state."Conti" ("Énum"), "errin"=w269, "test ok ?"=w271) -> ("errout"=w290:errorcluster, "Next"=w275:T5)  [unwired: 5 in]
      }
      frame "Conti" {
        w334 = i16 2 ("largeur (-)")
        # "Continuité des modules pour proto"
        n116 = global read "VG_BT3562.vi" "BT3562"() -> (w327:string)
        n117 = while {
          tunnel: w323 -> [w365]
          shift-right: [w361] -> _
          shift-left: _ -> [w363]
          tunnel: [w361] -> w332
          tunnel: w327 -> [w362]
          shift-right: [w358] -> _
          shift-left: _ -> [w360]
          tunnel: [w357] -> w328
          tunnel: [w356] -> w320
          stop <- w359 stop-if-true
          w357 = 5.0 ("y")
          n118 = call "QA.vi"("ERRIN"=w365, "VISA"=w362) -> ("ERROUT"=w356:errorcluster, "DATAOUT"=w364:string)  [unwired: 8 in]
          n119 = Fract/Exp String To Number(string=w364) -> (number=w353:dbl)  [unwired: 3 in, 1 out]
          n120 = In Range and Coerce(upper limit=1000000.0 ("limite supérieure"), x=w353, lower limit=0.0 ("limite inférieure")) -> (In Range?=w355:bool)  [unwired: 1 out]
          n121 = case shown="True" w355 {
            tunnel: w363 -> [_ w371]
            tunnel: [w366 w370] -> w361
            tunnel: w353 -> [_ w369]
            tunnel: w360 -> [_ w368]
            tunnel: [w366 w367] -> w358
            frame False {
              w366 = 0.0
            }
            frame True {
              n122 = Add(x=w369, y=w371) -> (x+y=w370:dbl)
              n123 = Increment(x=w368) -> (x+1=w367:dbl)
            }
          }
          n124 = Greater Or Equal?(x=w358, y=w357) -> (x >= y?=w359:bool)
        }
        n125 = call <userlib>:"FGV_Image.vi"("Énum"=FGV."SET", "IN"="CONTEST") -> ()  [unwired: 9 in, 1 out]
        n126 = local write "TOP"("Mesure de continuité" ("TOP")) -> ()
        n127 = Divide(x=w332, y=w328) -> (x/y=w326:dbl)
        n128 = Multiply(x=1000.0, y=w326) -> (x*y=w324:dbl)
        n129 = global read "OP500ZP_VGConf.vi" "Rmax"() -> (w333:dbl)
        n130 = Number To Fractional String(number=w324, width (-)=w334, precision (6)=w334) -> (F-format string=w335:string)  [unwired: 1 in]
        n131 = Less Or Equal?(x=w324, y=w333) -> (x <= y?=w341:bool)
        n132 = local read "BDD"() -> (w339:T1)
        n133 = Bundle By Name(cluster=w339, "Conti"=w335) -> (w338:T1)
        n134 = call "OP500ZP_LaunchLB.vi"("errin"=w320, "Application à lancer"=path "C:/Users/operateur/Desktop/FORSEE Diag tool V1.7.1/FORSEE_Diag.exe") -> ("error out"=w322:errorcluster)  [unwired: 7 in]
        n135 = local write "BDD"(w338) -> ()
        n136 = call "ZenPlusOP300_refaire.vi"("image"="Refaire", "refaire"=w342, "casOK"=OP500ZP_state."DTC", "errin"=w322, "test ok ?"=w341) -> ("errout"=w343:errorcluster, "Next"=w336:T5)  [unwired: 5 in]
        n137 = Concatenate Strings("Conti;" ("chaîne"), w335) -> (w351:string)
        n138 = call <userlib>:"Log_basic.vi"("errin"=w349, "date?"=TRUE, "chaîne"=w351, "in"=w348) -> ("sortie d'erreur"=w346:errorcluster, "refnum en sortie"=w347:refnum<file>)  [unwired: 6 in]
      }
      frame "DTC" {
        # "Chercher moyen de simplifier"
        # "Vérification de l'absence de DTC dans FDT"
        n139 = call "Multi_OUI_NON.vi"("errin"=w376, "errinb"=TRUE, "Tableau"=string[] ["FDTCHECK", "DTC1"]) -> ("errout"=w375:errorcluster, "isok?"=w374:bool)  [unwired: 7 in]
        n140 = case shown="True" w374 {
          tunnel: w375 -> [w408 w414]
          tunnel: [w408 w411] -> w383
          tunnel: [w407 w412] -> w382
          tunnel: [w407 w410] -> w378
          tunnel: [w407 w409] -> w379
          frame False {
            w407 = FALSE ("Aucun DTC")
          }
          frame True {
            n141 = call "Boîte de dialogue utilisateur"("Enable"=TRUE, "error in (no error)"=w414) -> ("Présence de DTC"=w409:bool, "Aucun DTC"=w410:bool, "OK"=w412:bool, "error out"=w411:errorcluster)  [unwired: 14 in]
            n142 = call "OUINON.vi"("image"="DTC2" ("IN")) -> ()  [unwired: 9 in, 2 out]
          }
        }
        n143 = And(x=w382, y=w378) -> (x .and. y?=w380:bool)
        n144 = case shown="False" w380 {
          selector: w380 -> [_ w421]
          tunnel: [w416 w420] -> w381
          tunnel: w379 -> [w417 w422]
          frame False {
            n145 = case shown="False" w417 {
              tunnel: [FALSE FALSE] -> w416
              frame False {
              }
              frame True {
              }
            }
          }
          frame True {
            n146 = case shown="True" w422 {
              tunnel: w421 -> [w423 _]
              tunnel: [w423 FALSE] -> w420
              frame False {
              }
              frame True {
              }
            }
          }
        }
        n147 = case shown="True" w381 {
          selector: w381 -> [w400 w403]
          tunnel: w383 -> [w401 w406]
          tunnel: [w401 w404] -> w397
          tunnel: [w400 w403] -> w372
          tunnel: [";DTC DETECTE(S)" "NO DTC;"] -> w385
          frame False {
          }
          frame True {
            n148 = call "OUINON.vi"("errin"=w406, "image"="DTC3" ("IN")) -> ("error out"=w404:errorcluster)  [unwired: 8 in, 1 out]
          }
        }
        n149 = Concatenate Strings("DTC;" ("chaîne"), w385) -> (w392:string)
        n150 = call <userlib>:"Log_basic.vi"("errin"=w389, "date?"=TRUE, "chaîne"=w392, "in"=w387) -> ("sortie d'erreur"=w388:errorcluster, "refnum en sortie"=w386:refnum<file>)  [unwired: 6 in]
        n151 = call "ZenPlusOP300_refaire.vi"("image"="Refaire", "refaire"=w395, "casOK"=OP500ZP_state."Next", "errin"=w397, "test ok ?"=w372) -> ("errout"=w396:errorcluster, "Next"=w393:T5)  [unwired: 5 in]
      }
      frame "DataDyn" {
        w426 = OP500ZP_state."DataDyn"  # Énum
        w435 = enum16{"STR", "DBL", "U32"}."DBL" ("Énum")
        w437 = "Vpack" ("section")
        # "tension du pack en sortie"
        n152 = call <userlib>:"Read_Param.vi"("Énum"=w435, "errin"=w439, "section"=w437, "key"="Min") -> ("error out"=w440:errorcluster, "dbl"=w433:dbl)  [unwired: 3 in, 3 out]
        n153 = call <userlib>:"Read_Param.vi"("Énum"=w435, "errin"=w440, "section"=w437, "key"="Max") -> ("error out"=w438:errorcluster, "dbl"=w434:dbl)  [unwired: 3 in, 3 out]
        n154 = call "OUINON.vi"("errin"=w438, "image"="Vpack" ("IN")) -> ("error out"=w442:errorcluster, "OUI/NON"=w430:bool)  [unwired: 8 in]
        n155 = case shown="True" w430 {
          selector: w430 -> [w449 _]
          tunnel: w442 -> [w451 w459]
          tunnel: [w451 w456] -> w443
          tunnel: ["ERR" w457] -> w428
          tunnel: [w449 w454] -> w429
          tunnel: w434 -> [_ w452]
          tunnel: w433 -> [_ w453]
          frame False {
          }
          frame True {
            w458 = i16 3 ("largeur (-)")
            n156 = call "Tension de l'étage bas"("error in (no error)"=w459) -> ("Vpack"=w455:dbl, "error out"=w456:errorcluster)  [unwired: 16 in, 1 out]
            n157 = In Range and Coerce(upper limit=w452, x=w455, lower limit=w453) -> (In Range?=w454:bool)  [unwired: 1 out]
            n158 = Number To Fractional String(number=w455, width (-)=w458, precision (6)=w458) -> (F-format string=w457:string)  [unwired: 1 in]
          }
        }
        n159 = Concatenate Strings("Vpack;" ("chaîne"), w428) -> (w431:string)
        n160 = call <userlib>:"Log_basic.vi"("errin"=w448, "chaîne"=w431, "in"=w447) -> ("sortie d'erreur"=w445:errorcluster, "refnum en sortie"=w446:refnum<file>)  [unwired: 7 in]
        n161 = call "OP500ZP_OuCrash.vi"("Booléen"=w429, "in"=w426) -> ("OUT"=w425:T5)  [unwired: 1 in]
      }
      frame "DataDyn2" {
        n162 = disable-structure shown="Désactivé" {
          disable-tunnel: [w508 _] -> w460
          disable-tunnel: w469 -> [w507 _]
          disable-tunnel: w468 -> [w506 _]
          disable-tunnel: w467 -> [w505 _]
          disable-tunnel: w465 -> [w504 _]
          disable-tunnel: [w503 _] -> w464
          disable-tunnel: [w502 _] -> w463
          disable-tunnel: [w501 _] -> w462
          disable-tunnel: w461 -> [w500 _]
          frame Disabled {
            w485 = OP500ZP_state."Demontage" ("Énum")
            n163 = property on="progression" class="Slide (strict)"(error in=w500, "Visible"=TRUE, "Value"=u8 0 ("progression")) -> (error out=w490:errorcluster)  [unwired: 1 in, 1 out]
            n164 = local write "TOP"("Analyse 2 des CMU ..." ("TOP")) -> ()
            n165 = flat-sequence {
              tunnel: [w520] -> w473
              tunnel: [w519] -> w499
              tunnel: [w518] -> w498
              tunnel: [w517] -> w497
              tunnel: [w516] -> w496
              tunnel: [w515] -> w495
              tunnel: w490 -> [w514]
              frame #0 {
                n166 = call "SCAN CMU.vi"("errin"=w514, "Nb modules"=i16 16) -> ("errout"=w520:errorcluster, "# température + #tension OK?"=w515:bool, "Vmin"=w519:dbl, "Vmax"=w518:dbl, "Tmin"=w516:dbl, "Tmax"=w517:dbl)  [unwired: 4 out]
                n167 = call <userlib>:"FGV_Image.vi"("Énum"=FGV."SET", "IN"="DataDyn") -> ()  [unwired: 9 in, 1 out]
              }
            }
            n168 = global read "IS30%.vi" "VG IS30% ?"() -> (w471:bool)
            n169 = call "OP400ZP_Test_DataDyn.vi"("Tcell Min (°C)"=w496, 1:w506, "is30%?"=w471, "MCU"=w495, "Tcell Max (°C)"=w497, "Température usine (°C)"=21.0, "errin"=w473, "testname"="Dyn2;", "Vcell Min (V)"=w499, "Vcell Max (V)"=w498) -> ("pass"=w472:bool, "datalog"=w510:string, "StrData"=w476:T10, "errout"=w474:errorcluster)  [unwired: 1 in, 1 out]
            n170 = Unbundle By Name(w476) -> ("Chaîne"=w481:string, "Chaîne"=w480:string, "Chaîne"=w479:string, "Chaîne"=w478:string, "Chaîne"=w477:string)
            n171 = call <userlib>:"Log_basic.vi"("errin"=w504, "date?"=TRUE, "chaîne"=w510, "in"=w505) -> ("sortie d'erreur"=w503:errorcluster, "refnum en sortie"=w502:refnum<file>)  [unwired: 6 in]
            n172 = local read "BDD"() -> (w483:T1)
            n173 = Bundle By Name(cluster=w483, "2_TCellmin"=w481, "2_TCellmax"=w480, "2_VCellmin"=w479, "2_VCellmax"=w478, "2_Nbmodule"=w477) -> (w482:T1)
            n174 = call "ZenPlusOP300_refaire.vi"("image"="Refaire", "refaire"=w507, "Pédale"=FALSE, "errin"=w474, "test ok ?"=w472) -> ("errout"=w486:errorcluster, "Next"=w508:T5, "casOK"=w470:T5)  [unwired: 4 in]
            n175 = local write "BDD"(w482) -> ()
            n176 = property on="progression" class="Slide (strict)"(error in=w486, "Visible"=FALSE, "Value"=u8 0 ("progression")) -> (error out=w501:errorcluster)  [unwired: 1 in, 1 out]
          }
          frame Enabled {
          }
        }
      }
      frame "Crash" {
        # "\\\\forseepower.com\\fr\\040 Production\\FR7 - Poitiers\\06 Production\\05. Electronique\\Documents Control lib\\Archives\\ZEN PLUS"
        n177 = Close File(refnum=w546, error in=w545) -> (path=w536:path, error out=w539:errorcluster)
        n178 = call <userlib>:"FGV_Image.vi"("Énum"=FGV."SET", "IN"="TeamLeader") -> ()  [unwired: 9 in, 1 out]
        n179 = case shown="No Error" w523 {
          selector: w523 -> [w551 w552]
          tunnel: [w551 w552] -> w522
          frame No Error {
            n180 = local read "BDD"() -> (w549:T1)
            n181 = Bundle By Name(cluster=w549, "PASS"="0") -> (w550:T1)
            n182 = local write "BDD"(w550) -> ()
          }
          frame Error {
          }
        }
        n183 = call <userlib>:"waitXms.vi"("attente (ms)"=u32 500, "errin"=w539) -> ("errout"=w537:errorcluster)  [unwired: 13 in]
        n184 = Read from Text File(file (use dialog)=w536, error in=w537) -> (text=w535:string, error out=w533:errorcluster)  [unwired: 2 in, 2 out]
        n185 = call "OP500ZP_SN_Reader.vi"("Fichier txt"=w535) -> ("SN"=w528:string)  [unwired: 10 in]
        n186 = local read "BDD"() -> (w530:T1)
        n187 = Unbundle By Name(w530) -> ("PN"=w527:string)
        n188 = Concatenate Strings(w527, "-SN" ("chaîne"), w528) -> (w529:string)
        n189 = call "OP500ZP_NouveauDossier.vi"("entrée d'erreur (pas d'erreur)"=w533, "Nom du repertoire (PN SN)"=w529, "Network before adding a new folder"=path "\\\\forseepower.com\\fr/040 Production/FR7 - Poitiers/06 Production/05. Electronique/Documents Control lib/Archives/ZEN PLUS" ("chemin de la cible (utiliser une boîte de dialogue)")) -> ("sortie d'erreur"=w534:errorcluster, "Network after adding a new folder"=w531:path)  [unwired: 7 in]
        n190 = local read "BDD"() -> (w521:T1)
        n191 = Copy ("Copier")(8:w534, 10:w531, 11:w536) -> (0:w538:errorcluster)  [unwired: 2 in, 2 out]
        n192 = call "PvgeneratorOP500.vi"("errin"=w538, "BDD"=w521, "network"=w531, "path in"=w536) -> ("sortie d'erreur"=w542:errorcluster, "network out"=w541:path)  [unwired: 4 in, 2 out]
        n193 = call <userlib>:"POP_GOOGLE.vi"("error in"=w542, "chemin"=w541) -> ("error out"=w524:errorcluster)  [unwired: 8 in, 1 out]
        n194 = flat-sequence {
          tunnel: [TRUE] -> w547
          tunnel: w524 -> [_]
          frame #0 {
          }
        }
      }
      frame "Next" {
        w576 = OP500ZP_state."Null"  # Énum
        w577 = OP500ZP_state."Scan"  # Énum
        # "\\\\forseepower.com\\fr\\040 Production\\FR7 - Poitiers\\06 Production\\05. Electronique\\Documents Control lib\\Archives\\ZEN PLUS"
        n195 = Close File(refnum=w579, error in=w578) -> (path=w559:path, error out=w575:errorcluster)
        n196 = call <userlib>:"waitXms.vi"("attente (ms)"=u32 500, "errin"=w575) -> ("errout"=w571:errorcluster)  [unwired: 13 in]
        n197 = Read from Text File(file (use dialog)=w559, error in=w571) -> (text=w569:string, error out=w568:errorcluster)  [unwired: 2 in, 2 out]
        n198 = case shown="No Error" w555 {
          selector: w555 -> [w585 w586]
          tunnel: [w585 w586] -> w554
          frame No Error {
            n199 = local read "BDD"() -> (w583:T1)
            n200 = Bundle By Name(cluster=w583, "PASS"="1") -> (w584:T1)
            n201 = local write "BDD"(w584) -> ()
          }
          frame Error {
          }
        }
        n202 = call "OP500ZP_SN_Reader.vi"("Fichier txt"=w569) -> ("SN"=w561:string)  [unwired: 10 in]
        n203 = local read "BDD"() -> (w564:T1)
        n204 = Unbundle By Name(w564) -> ("PN"=w563:string)
        n205 = call "OUINON.vi"("errin"=w554, "image"="Next" ("IN")) -> ("error out"=w558:errorcluster, "OUI/NON"=w580:bool)  [unwired: 8 in]
        n206 = Concatenate Strings(w563, "-SN" ("chaîne"), w561) -> (w560:string)
        n207 = call "OP500ZP_NouveauDossier.vi"("entrée d'erreur (pas d'erreur)"=w568, "Nom du repertoire (PN SN)"=w560, "Network before adding a new folder"=path "\\\\forseepower.com\\fr/040 Production/FR7 - Poitiers/06 Production/05. Electronique/Documents Control lib/Archives/ZEN PLUS" ("chemin de la cible (utiliser une boîte de dialogue)")) -> ("sortie d'erreur"=w567:errorcluster, "Network after adding a new folder"=w565:path)  [unwired: 7 in]
        n208 = Select(t=w577, s=w580, f=w576) -> (s? t:f=w557:T5)
        n209 = Copy ("Copier")(8:w567, 10:w565, 11:w559) -> (0:w570:errorcluster)  [unwired: 2 in, 2 out]
        n210 = call "PvgeneratorOP500.vi"("errin"=w570, "network"=w565, "path in"=w559) -> ("sortie d'erreur"=w573:errorcluster, "network out"=w572:path)  [unwired: 5 in, 2 out]
        n211 = call <userlib>:"POP_GOOGLE.vi"("error in"=w573, "chemin"=w572) -> ("error out"=w556:errorcluster)  [unwired: 8 in, 1 out]
      }
      frame "Comext" {
        n212 = disable-structure shown="Désactivé" {
          disable-tunnel: w597 -> [w611 _]
          disable-tunnel: w596 -> [w610 _]
          disable-tunnel: [w609 _] -> w595
          disable-tunnel: w594 -> [w608 _]
          disable-tunnel: [w607 _] -> w593
          disable-tunnel: w592 -> [w606 _]
          disable-tunnel: w591 -> [w604 _]
          disable-tunnel: [w602 _] -> w590
          disable-tunnel: w589 -> [w601 _]
          disable-tunnel: [w599 _] -> w588
          disable-tunnel: [w598 _] -> w587
          frame Disabled {
            n213 = call "OUINON.vi"("errin"=w604, "image"="Comext" ("IN")) -> ("error out"=w603:errorcluster, "OUI/NON"=w600:bool)  [unwired: 8 in]
            n214 = case shown="True" w600 {
              tunnel: w611 -> [w616 w628]
              tunnel: w610 -> [w615 w627]
              tunnel: [w615 w626] -> w599
              tunnel: [w616 w625] -> w609
              tunnel: [OP500ZP_state."Crash" ("OUT") w624] -> w598
              tunnel: w608 -> [_ w623]
              tunnel: [w613 w622] -> w607
              tunnel: w606 -> [_ w621]
              tunnel: w603 -> [w613 w620]
              tunnel: [w614 w619] -> w602
              tunnel: w601 -> [w614 w619]
              frame False {
              }
              frame True {
                (unwired) "Comext;" ("testname")
                (unwired) OP500ZP_state."Demontage"  # Énum
                n215 = local read "PN"() -> (w639:string)
                n216 = call <vilib>:"Application Directory.vi"() -> ("Application Directory"=w641:path)
                n217 = call <userlib>:"Read_Param.vi"("Énum"=enum16{"STR", "DBL", "U32"}."U32", "errin"=w620, 9:w641, "section"="DataDyn", "key"=w639) -> ("error out"=w634:errorcluster, "U32"=w637:u32)  [unwired: 2 in, 3 out]
                n218 = call <userlib>:"FGV_Image.vi"("Énum"=FGV."SET", "IN"="DataDyn") -> ()  [unwired: 9 in, 1 out]
                n219 = property on="progression" class="Slide (strict)"(error in=w634, "Visible"=TRUE, "Value"=u8 0 ("progression")) -> (error out=w633:errorcluster)  [unwired: 1 in, 1 out]
                n220 = call "SCAN CMU.vi"("errin"=w633, "Nb modules"=w637) -> ("errout"=w651:errorcluster, "# température + #tension OK?"=w646:bool, "Vmin"=w650:dbl, "Vmax"=w649:dbl, "Tmin"=w647:dbl, "Tmax"=w648:dbl)  [unwired: 4 out]
                n221 = call "OP500ZP_Test_DataDyn.vi"("Vcell Max (V)"=w649, "MCU"=w646, "Vcell Min (V)"=w650, "appdir"=w621, "errin"=w651, "Température usine (°C)"=21.0, "Tcell Max (°C)"=w648, "Tcell Min (°C)"=w647) -> ("errout"=w645:errorcluster, "datalog"=w653:string, "pass"=w644:bool)  [unwired: 1 out]
                n222 = call <userlib>:"Log_basic.vi"("errin"=w628, "date?"=TRUE, "chaîne"=w653, "in"=w627) -> ("sortie d'erreur"=w625:errorcluster, "refnum en sortie"=w626:refnum<file>)  [unwired: 6 in]
                n223 = call "ZenPlusOP300_refaire.vi"("image"="Refaire", "refaire"=w623, "Pédale"=FALSE, "errin"=w645, "test ok ?"=w644) -> ("errout"=w629:errorcluster, "Next"=w624:T5)  [unwired: 5 in]
                n224 = property on="progression" class="Slide (strict)"(error in=w629, "Visible"=FALSE, "Value"=u8 0 ("progression")) -> (error out=w622:errorcluster)  [unwired: 1 in, 1 out]
              }
            }
          }
          frame Enabled {
          }
        }
      }
      frame "MCU" {
        # "GetProcessHandleFromWindowTitle"
        # "v"
        # "Fermer FDT"
        n225 = call "OUINON.vi"("errin"=w691, "image"="FDTPREMCU1") -> ("error out"=w672:errorcluster, "OUI/NON"=w673:bool)  [unwired: 8 in]
        n226 = call "Boite.vi"("Enable"=w673, "error in (no error)"=w672) -> ("Température usine"=w669:dbl, "Nombre de température"=w670:dbl, "Nombre de tensons"=w671:dbl, "error out"=w667:errorcluster)  [unwired: 13 in, 1 out]
        n227 = local write "TOP"("Mesure MCU" ("TOP")) -> ()
        n228 = global read "PackType.vi" "VG_PackType"() -> (w689:string)
        n229 = call "OUINON.vi"("errin"=w667, "image"="EXIT") -> ("error out"=w666:errorcluster, "OUI/NON"=w665:bool)  [unwired: 8 in]
        n230 = case shown="\"ZEN77\"" w689 {
          tunnel: w670 -> [_ w722 w731 w735 w742 w750]
          tunnel: [FALSE w721 w728 w736 w743 w749] -> w679
          tunnel: w671 -> [_ w720 w727 w734 w741 w748]
          tunnel: [0.0 ("ZEN84TEMP") w719 w726 w733 w740 w747] -> w677
          tunnel: [0.0 ("ZEN84TENS") w718 w725 w732 w739 w746] -> w675
          frame "Faux", Default {
          }
          frame "ZEN74" {
            n231 = global read "OP500ZP_VGConf.vi" "ZEN74TENS"() -> (w718:dbl)
            n232 = global read "OP500ZP_VGConf.vi" "ZEN74TEMP"() -> (w719:dbl)
            n233 = Equal?(x=w722, y=w719) -> (x = y?=w723:bool)
            n234 = Equal?(x=w720, y=w718) -> (x = y?=w724:bool)
            n235 = And(x=w723, y=w724) -> (x .and. y?=w721:bool)
          }
          frame "ZEN77" {
            n236 = global read "OP500ZP_VGConf.vi" "ZEN77TENS"() -> (w725:dbl)
            n237 = global read "OP500ZP_VGConf.vi" "ZEN77TEMP"() -> (w726:dbl)
            n238 = Equal?(x=w731, y=w726) -> (x = y?=w729:bool)
            n239 = Equal?(x=w727, y=w725) -> (x = y?=w730:bool)
            n240 = And(x=w729, y=w730) -> (x .and. y?=w728:bool)
          }
          frame "ZEN79" {
            n241 = global read "OP500ZP_VGConf.vi" "ZEN79TENS"() -> (w732:dbl)
            n242 = global read "OP500ZP_VGConf.vi" "ZEN79TEMP"() -> (w733:dbl)
            n243 = Equal?(x=w735, y=w733) -> (x = y?=w737:bool)
            n244 = Equal?(x=w734, y=w732) -> (x = y?=w738:bool)
            n245 = And(x=w737, y=w738) -> (x .and. y?=w736:bool)
          }
          frame "ZEN82" {
            n246 = global read "OP500ZP_VGConf.vi" "ZEN82TENS"() -> (w739:dbl)
            n247 = global read "OP500ZP_VGConf.vi" "ZEN82TEMP"() -> (w740:dbl)
            n248 = Equal?(x=w742, y=w740) -> (x = y?=w744:bool)
            n249 = Equal?(x=w741, y=w739) -> (x = y?=w745:bool)
            n250 = And(x=w744, y=w745) -> (x .and. y?=w743:bool)
          }
          frame "ZEN84" {
            n251 = global read "OP500ZP_VGConf.vi" "ZEN84TENS"() -> (w746:dbl)
            n252 = global read "OP500ZP_VGConf.vi" "ZEN84TEMP"() -> (w747:dbl)
            n253 = Equal?(x=w750, y=w747) -> (x = y?=w751:bool)
            n254 = Equal?(x=w748, y=w746) -> (x = y?=w752:bool)
            n255 = And(x=w751, y=w752) -> (x .and. y?=w749:bool)
          }
        }
        n256 = To Word Integer(number=w677) -> (16bit integer=w676:i16)
        n257 = To Word Integer(number=w675) -> (16bit integer=w674:i16)
        n258 = case shown="True" w665 {
          tunnel: [w707 w714] -> w692
          tunnel: ["0" ("Log") w713] -> w688
          tunnel: [FALSE ("is OK?") w712] -> w680
          tunnel: w669 -> [_ w711]
          tunnel: w666 -> [w707 w710]
          tunnel: [T8 {"", "", "", "", "", "", "", ""} ("ToBDD") w709] -> w664
          frame False {
          }
          frame True {
            n259 = call "OP500ZP_FDT_V2.vi"("errin"=w710, "TempUsine"=w711) -> ("errout"=w714:errorcluster, "Log"=w713:string, "is OK?"=w712:bool, "ToBDD"=w709:T8)  [unwired: 6 in]
          }
        }
        n260 = Number To Fractional String(number=w674, precision (6)=i16 0 ("précision (6)")) -> (F-format string=w681:string)  [unwired: 2 in]
        n261 = Number To Fractional String(number=w676, precision (6)=i16 0 ("précision (6)")) -> (F-format string=w683:string)  [unwired: 2 in]
        n262 = And(x=w680, y=w679) -> (x .and. y?=w678:bool)
        n263 = call "ZenPlusOP300_refaire.vi"("image"="Refaire", "refaire"=w694, "casOK"=OP500ZP_state."OCVACIR", "errin"=w692, "test ok ?"=w678) -> ("errout"=w696:errorcluster, "Next"=w693:T5)  [unwired: 5 in]
        n264 = Concatenate Strings(w688, ";TEMPERATURES;" ("chaîne"), w683, ";TENSIONS;" ("chaîne"), w681) -> (w685:string)
        n265 = Unbundle(w664) -> (w661:string, w660:string, w659:string, w658:string, w657:string, w656:string, w655:string, w654:string)
        n266 = call <userlib>:"Log_basic.vi"("errin"=w703, "date?"=TRUE, "chaîne"=w685, "in"=w702) -> ("sortie d'erreur"=w701:errorcluster, "refnum en sortie"=w700:refnum<file>)  [unwired: 6 in]
        n267 = local read "BDD"() -> (w663:T1)
        n268 = Bundle By Name(cluster=w663, "Ubatt"=w661, "1_DeltaV"=w660, "1_DeltaT"=w659, "1_TCellmax"=w658, "1_TCellmin"=w657, "1_VCellmax"=w656, "1_VCellmin"=w655, "TUsine"=w654) -> (w662:T1)
        n269 = local write "BDD"(w662) -> ()
      }
    }
    n270 = Wait (ms)(milliseconds to wait=u32 200 ("attente (ms)")) -> ()  [unwired: 1 out]
    n271 = case shown="False" w21 {
      selector: w21 -> [_ w753]
      frame False {
      }
      frame True {
        n272 = local write "STOP"(w753) -> ()
      }
    }
  }
  n273 = while {
    shift-right: [w762] -> _
    shift-left: errorcluster {"status"=FALSE, "code"=0, "source"=""} ("error out") -> [w759]
    stop <- w760 stop-if-true
    # "ici tu mets l'image à jour si besoin"
    n274 = Wait (ms)(milliseconds to wait=u32 100 ("attente (ms)")) -> ()  [unwired: 1 out]
    n275 = call <userlib>:"FGV_Image.vi"("Énum"=FGV."GET") -> ("OUT"=w755:string)  [unwired: 10 in]
    n276 = Not Equal?(x=w755, y="") -> (x != y?=w756:bool)
    n277 = case shown="True" w756 {
      tunnel: [w764 w769] -> w762
      tunnel: w759 -> [w764 w768]
      tunnel: w755 -> [_ w767]
      frame False {
      }
      frame True {
        n278 = call <vilib>:"Application Directory.vi"() -> ("Application Directory"=w772:path)
        n279 = Path To String(path=w772) -> (string=w773:string)
        n280 = Concatenate Strings(w773, "\\Image\\" ("chaîne"), w767, ".jpg" ("chaîne")) -> (w771:string)
        n281 = call <userlib>:"FGV_Image.vi"("Énum"=FGV."RAZ") -> ()  [unwired: 10 in, 1 out]
        n282 = String To Path(string=w771) -> (path=w770:path)
        n283 = call <vilib>:"Read JPEG File.vi"("error in (no error)"=w768, "path to JPEG file"=w770) -> ("error out"=w769:errorcluster, "image data"=w776:T11)  [unwired: 7 in, 1 out]
        n284 = call <vilib>:"Draw Flattened Pixmap.vi"("image data"=w776) -> ("new picture"=w765:picture)  [unwired: 8 in]
        n285 = local write "DRAW"(w765) -> ()
      }
    }
    n286 = global read "VG_progressBar.vi" "progression"() -> (→"progression":dbl)
    n287 = local read "STOP"() -> (w761:bool)
    n288 = Or(x=w762, y=w761) -> (x .or. y?=w760:bool)
  }
  n289 = while {
    tunnel: [w777] -> w2
    shift-right: [w778] -> _
    shift-left: errorcluster {"status"=FALSE, "code"=0, "source"=""} ("error out") -> [w778]
    stop <- w777 stop-if-true
    n290 = call "ARRET.vi"("arrêt"="?") -> ("T button?"=w777:bool)  [unwired: 10 in]
  }
  n291 = Stop(stop? (T)=w2) -> ()
  n292 = Merge Errors(w19, w18) -> (→"errout":errorcluster)
  n293 = disable-structure shown="Activé" {
    disable-tunnel: [w780 _] -> _
    frame Disabled {
      n294 = call "Data Dynamiques"() -> ("CMU OK"=w780:bool)  [unwired: 12 in, 7 out]
    }
    frame Enabled {
    }
  }
  "STOP" <- w16
